vi "Variant to Array.vi"(8 "error in (no error)":errorcluster, 11 "value":variant) -> (0 "error out":errorcluster, 3 "Array":dbl[](array[numeric]))   [LabVIEW 2016, in "LVtoITX.lvclass"]
uses:
  LVtoITX.lvclass
  <vilib>/Utility/Data Type/NI_Data Type.lvlib
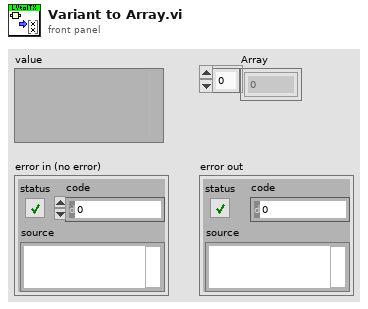
[diagram p1: front panel]
types:
  T1 = typedef "NI_Data Type.lvlib/Data Type.ctl" = enum8{"Invalid Type", "Void", "I8", "I16", "I32", "I64", "U8", "U16", "U32", "U64", "Single Float", "Double Float", "Extended Float", "Single Complex", "Double Complex", "Extended Complex", "Enum U8", "Enum U16", "Enum U32", "Enum U64", "Single Float With Unit", "Double Float With Unit", "Extended Float With Unit", "Single Complex with Unit", "Double Complex with Unit", "Extended Complex with Unit", "Boolean", "String", "Path", "Picture", "Tag", "Array", "Cluster", "Variant", "LV Variant", "Waveform", "Timestamp", "Digital Waveform", "Digital Data", "ExpressData", "Refnum", "External Data", "VI", "Poly VI", "LabVIEW Class Instance", "Fixed Point"}
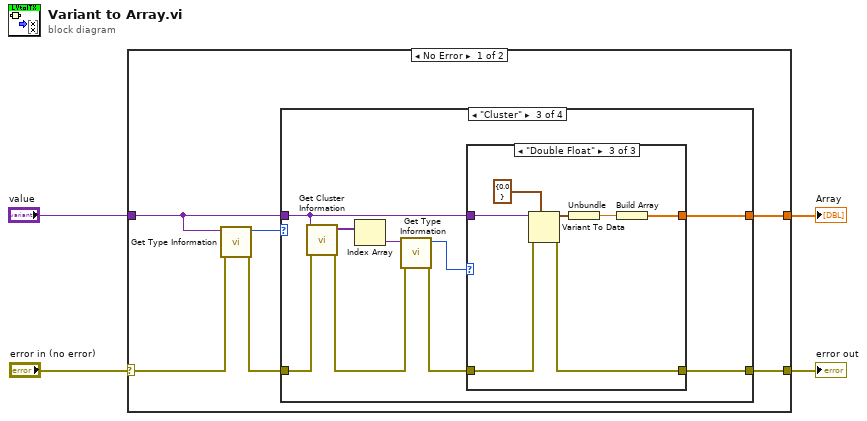
[diagram p0: block diagram]
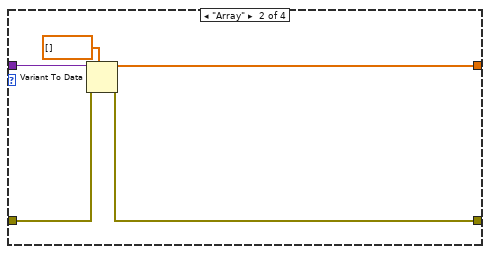
[diagram p3: hidden frame]
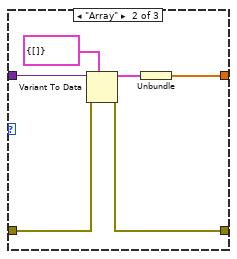
[diagram p5: hidden frame]
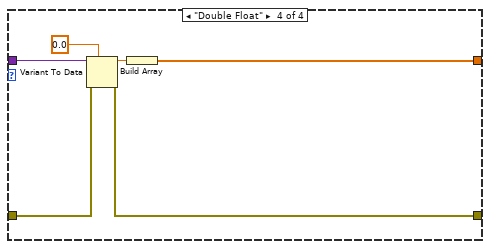
[diagram p6: hidden frame]
diagram:
  n1 = case shown="No Error" "error in (no error)" {
    selector: "error in (no error)" -> [w5 w46]
    tunnel: [w9 _] -> w4
    tunnel: [w6 w46] -> w3
    tunnel: "value" -> [w8 _]
    frame No Error {
      n2 = call <vilib>:"Get Type Information.vi"("error in (no error)"=w5, "Variant"=w8) -> ("error out"=w7:errorcluster, "Type"=w10:T1)  [unwired: 5 in, 3 out]
      n3 = case shown="\"Cluster\"" w10 {
        tunnel: [w11 w12 w20 w40] -> w6
        tunnel: [_ w15 w17 w42] -> w9
        tunnel: w8 -> [_ w14 w18 w44]
        tunnel: w7 -> [w11 w13 w25 w41]
        frame Default {
        }
        frame "Array" {
          n4 = Variant To Data(error in=w13, type=dbl[] [], Variant=w14) -> (data=w15:dbl[], error out=w12:errorcluster)
        }
        frame "Cluster" {
          n5 = call <vilib>:"Get Cluster Information.vi"("error in (no error)"=w25, "Variant"=w18) -> ("error out"=w22:errorcluster, "Cluster Elements"=w24:variant[])  [unwired: 8 in]
          n6 = Index Array(array=w24) -> (element=w23:variant)  [unwired: 1 in]
          n7 = call <vilib>:"Get Type Information.vi"("error in (no error)"=w22, "Variant"=w23) -> ("error out"=w21:errorcluster, "Type"=w19:T1)  [unwired: 5 in, 3 out]
          n8 = case shown="\"Double Float\"" w19 {
            tunnel: [w26 w30 w36] -> w20
            tunnel: [_ w28 w38] -> w17
            tunnel: w21 -> [w26 w31 w37]
            tunnel: w18 -> [_ w27 w33]
            frame Default {
            }
            frame "Array" {
              n9 = Variant To Data(error in=w31, type=cluster{dbl[]} {[]}, Variant=w27) -> (data=w32:cluster{dbl[]}, error out=w30:errorcluster)
              n10 = Unbundle(w32) -> (w28:dbl[])
            }
            frame "Double Float" {
              n11 = Variant To Data(error in=w37, type=cluster{dbl} {0.0}, Variant=w33) -> (data=w39:cluster{dbl}, error out=w36:errorcluster)
              n12 = Unbundle(w39) -> (w34:dbl)
              n13 = Build Array(w34) -> (w38:dbl[])
            }
          }
        }
        frame "Double Float" {
          n14 = Variant To Data(error in=w41, type=0.0, Variant=w44) -> (data=w45:dbl, error out=w40:errorcluster)
          n15 = Build Array(w45) -> (w42:dbl[])
        }
      }
    }
    frame Error {
    }
  }
  "Array" <- w4
  "error out" <- w3
